vi "Write Iteration.vi"(8 "error in (no error)":errorcluster, 10 "Iteration":i32, 11 "Attack in":refnum<class "Net Attack.lvclass">) -> (0 "error out":errorcluster, 3 "Attack out":refnum<class "Net Attack.lvclass">)   [LabVIEW 2014, in "Net Attack.lvclass"]
uses:
  Net Attack.lvclass
  Net Attack.lvclass/Net Attack.ctl
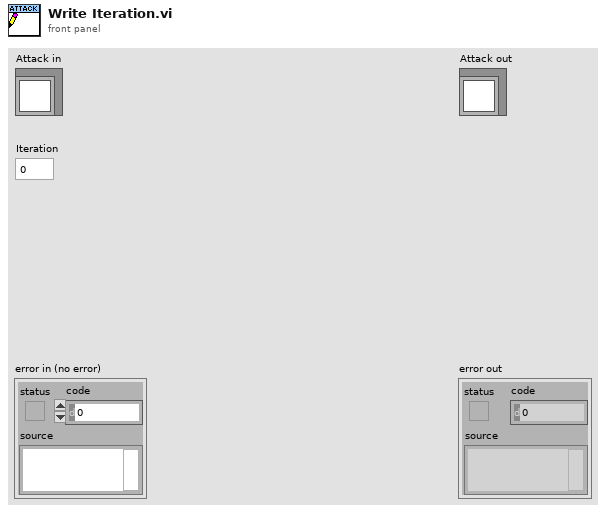
[diagram p1: front panel]
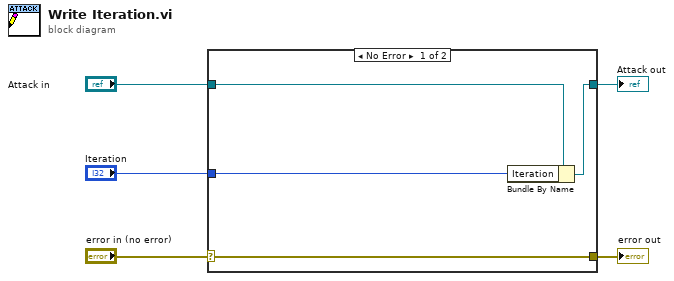
[diagram p0: block diagram]
diagram:
  n1 = case shown="No Error" "error in (no error)" {
    selector: "error in (no error)" -> [w9 w10]
    tunnel: [w9 w10] -> w4
    tunnel: [w7 w11] -> w2
    tunnel: "Attack in" -> [w8 w11]
    tunnel: "Iteration" -> [w6 _]
    frame No Error {
      n2 = Bundle By Name(cluster=w8, "Iteration"=w6) -> (w7:refnum<class "Net Attack.lvclass">)
    }
    frame Error {
    }
  }
  "error out" <- w4
  "Attack out" <- w2
